vi "c DMC60C get F.vi"(8 "error in (no error)":errorcluster, 10 "slot":i32, 11 "DMC60DevRef":T1={"DeviceStatus"={"status"=FALSE, "code"=0, "source"=""}, "Type"=enum."PWM", "PWM"={"PWM Channel"=enum."Invalid", "DeadBand"={"Name"="", "maxPositivePwm"=0, "minPositivePwm"=0, "centerPwm"=0, "maxNegativePwm"=0, "minNegativePwm"=0, "angularRange"=0}}, "CAN"={"Device Number"=0, "SetOutput VI Ref"=variant, "GetOutput VI Ref"=variant, "Enable VI Ref"=variant, "Disable VI Ref"=variant, "Data"=variant}, "Invert"=FALSE, "DIO PWM"={"PWM \"Enable\" Channel"=enum."Invalid", "DIOChannel"=enum."Invalid", "PWM Rate"=0.0}}) -> (0 "error out":errorcluster, 2 "function return":sgl, 3 "DMC60DevRef":T1={"DeviceStatus"={"status"=FALSE, "code"=0, "source"=""}, "Type"=enum."PWM", "PWM"={"PWM Channel"=enum."Invalid", "DeadBand"={"Name"="", "maxPositivePwm"=0, "minPositivePwm"=0, "centerPwm"=0, "maxNegativePwm"=0, "minNegativePwm"=0, "angularRange"=0}}, "CAN"={"Device Number"=0, "SetOutput VI Ref"=variant, "GetOutput VI Ref"=variant, "Enable VI Ref"=variant, "Disable VI Ref"=variant, "Data"=variant}, "Invert"=FALSE, "DIO PWM"={"PWM \"Enable\" Channel"=enum."Invalid", "DIOChannel"=enum."Invalid", "PWM Rate"=0.0}})   [LabVIEW 2018, in "DMC60C.lvlib"]
doc: "float c_getF(int dev, unsigned int slot);"
uses:
  <vilib>/Rock Robotics/WPI/ThirdParty/TopLevel/DMC60C/DMC60C.lvlib
  <vilib>/Rock Robotics/WPI/MotorControl/WPI_MotorControlDeviceRef.ctl
  <vilib>/Rock Robotics/WPI/MotorControl/WPI_MotorControlType.ctl
  <vilib>/Rock Robotics/SystemInterfaces/DIO/FPGA_DIOPWMChannel.ctl
  <vilib>/Rock Robotics/WPI/PWM/WPI_PWMDeadband.ctl
  <vilib>/Rock Robotics/SystemInterfaces/DIO/FPGA_DIOChannel.ctl
  <vilib>/Rock Robotics/WPI/ThirdParty/TopLevel/DMC60C/DMC60CDeviceRef.ctl
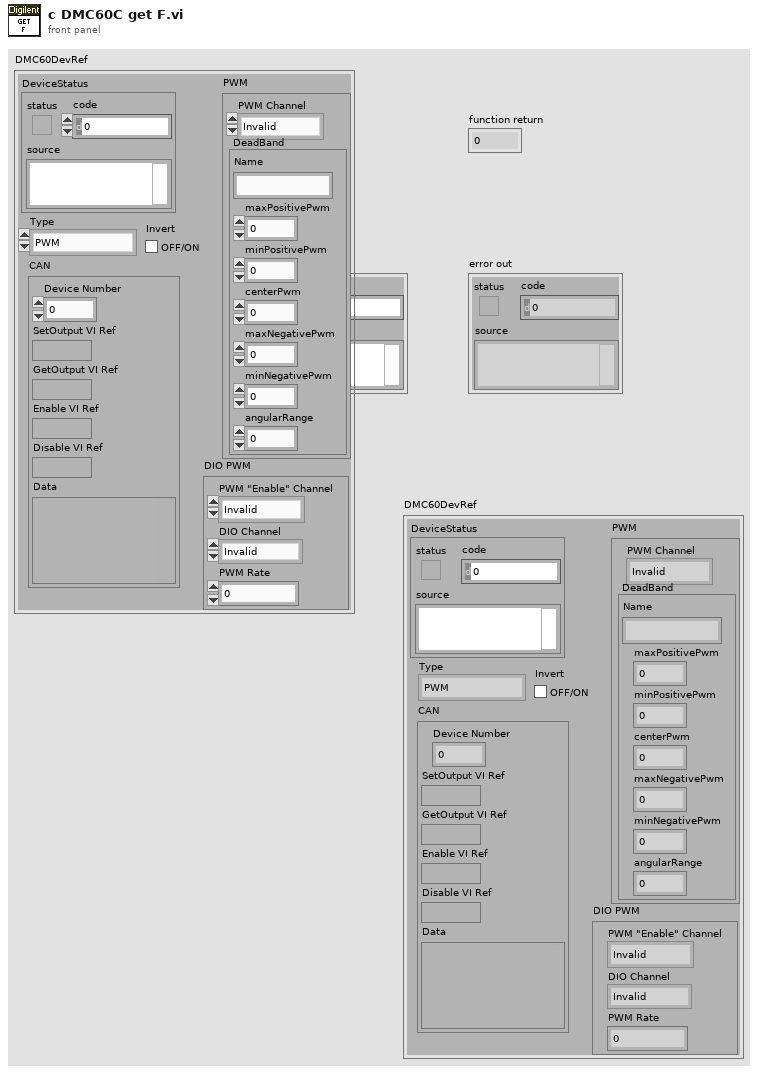
[diagram p1: front panel]
types:
  T1 = typedef "WPI_MotorControlDeviceRef.ctl" = cluster{"DeviceStatus":errorcluster, "Type":T2, "PWM":cluster{"PWM Channel":T3, "DeadBand":T4}, "CAN":cluster{"Device Number":u8, "SetOutput VI Ref":variant, "GetOutput VI Ref":variant, "Enable VI Ref":variant, "Disable VI Ref":variant, "Data":variant}, "Invert":bool, "DIO PWM":cluster{"PWM \"Enable\" Channel":T3, "DIOChannel":T5, "PWM Rate":dbl}}
  T2 = typedef "WPI_MotorControlType.ctl" = enum16{"PWM", "CAN", "DIO PWM"}
  T3 = typedef "FPGA_DIOPWMChannel.ctl" = enum8{"PWM 0", "PWM 1", "PWM 2", "PWM 3", "PWM 4", "PWM 5", "PWM 6", "PWM 7", "PWM 8", "PWM 9", "PWM MXP 0", "PWM MXP 1", "PWM MXP 2", "PWM MXP 3", "PWM MXP 4", "PWM MXP 5", "PWM MXP 6", "PWM MXP 7", "PWM MXP 8", "PWM MXP 9", "Invalid"}
  T4 = typedef "WPI_PWMDeadband.ctl" = cluster{"Name":string, "maxPositivePwm":i32, "minPositivePwm":i32, "centerPwm":i32, "maxNegativePwm":i32, "minNegativePwm":i32, "angularRange":u16}
  T5 = typedef "FPGA_DIOChannel.ctl" = enum8{"DIO 0", "DIO 1", "DIO 2", "DIO 3", "DIO 4", "DIO 5", "DIO 6", "DIO 7", "DIO 8", "DIO 9", "DIO MXP 0", "DIO MXP 1", "DIO MXP 2", "DIO MXP 3", "DIO MXP 4", "DIO MXP 5", "DIO MXP 6", "DIO MXP 7", "DIO MXP 8", "DIO MXP 9", "DIO MXP 10", "DIO MXP 11", "DIO MXP 12", "DIO MXP 13", "DIO MXP 14", "DIO MXP 15", "SPI Port CS1", "SPI Port CS2", "SPI Port CS3", "SPI Port MISO", "SPI Port MOSI", "Invalid"}
  T6 = typedef "DMC60C.lvlib/DMC60CDeviceRef.ctl" = cluster{"DeviceRef":i32, "arbID":u32}
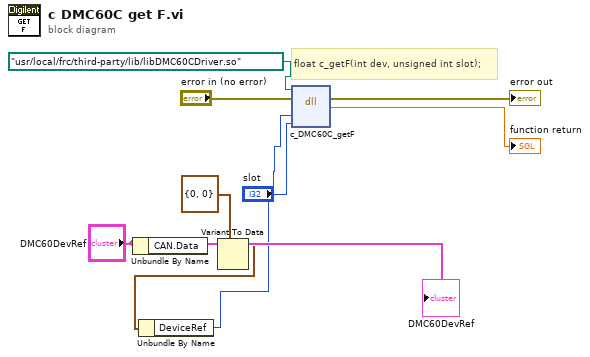
[diagram p0: block diagram]
diagram:
  # "float c_getF(int dev, unsigned int slot);"
  n1 = Unbundle By Name("DMC60DevRef") -> ("CAN.Data"=w5:variant)
  n2 = Variant To Data(type=T6 {"DeviceRef"=0, "arbID"=0} ("DMC60C Device Ref"), Variant=w5) -> (data=w3:T6)  [unwired: 1 in, 1 out]
  n3 = Unbundle By Name(w3) -> ("DeviceRef"=w2:i32)
  n4 = dll-call lib="usr/lib/libdmc60c.so" fn="c_DMC60C_getF"(path in=path "/usr/local/frc/third-party/lib/libDMC60CDriver.so", error in="error in (no error)", "dev"=w2, "slot"="slot") -> (error out=→"error out":errorcluster, "return type"=→"function return":sgl)  [unwired: 3 in, 1 out]
  "DMC60DevRef" <- "DMC60DevRef"
